vi "XIPIN_Floating-point_6_1.vi"   [LabVIEW 2017]
doc: "The Xilinx Floating-Point Operator is capable of being configured to provide a range of floating-point operations. The core offers addition, subtraction, multiplication, division, reciprocal, square-root, reciprocal-square-root, absolute value, logarithm, compare and conversion operations. High-speed, single-cycle throughput is provided at a wide range of wordlengths that includes both single and double precision. XtremeDSP slices can be used with certain operations.\n------------------------------------\n<b>Need License</b> : No\n<b>Interface</b> : AXI4-Stream"
uses:
  <vilib>/rvi/XilinxIP/XIPIN_XNode/niFpgaXIPIN.xnode
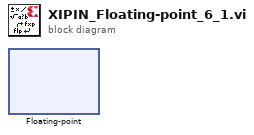
[diagram p0: block diagram]
diagram:
  n1 = xnode ("Floating-point")() -> ()
